vi "Add Logging Group - Right Click.vi"() -> ()   [LabVIEW 2015, in "Waveform Data Logger System Explorer.lvlib"]
uses:
  Waveform Data Logger System Explorer.lvlib
  <vilib>/NI Veristand/Custom Device API/Custom Device Item Ref.ctl
  Shared/Globals/Global GUIDs.vi
  <vilib>/NI VeriStand/Custom Device API/Custom Device API.lvlib
  Shared/Waveform Data Logger Shared.lvlib
panel:
  in  "Node Ptr":T1 format="%.0x"
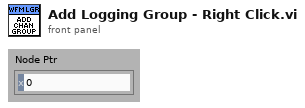
[diagram p1: front panel]
types:
  T1 = typedef "Custom Device API.lvlib/Custom Device Item Ref.ctl" = u64
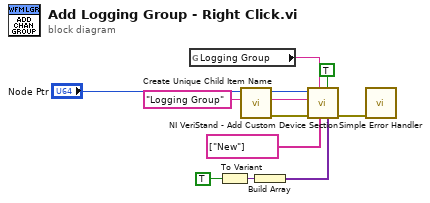
[diagram p0: block diagram]
diagram:
  n1 = global read "Global GUIDs.vi" "Logging Group"() -> (w8:string)
  n2 = To Variant(anything=TRUE) -> (Variant=w4:variant)
  n3 = call "Create Unique Child Item Name.vi"("Name in"="Logging Group", "Parent Item Ref in"="Node Ptr") -> ("error out"=w7:errorcluster, "Unique Name out"=w10:string, "Parent Item Ref out"=w11:T1)  [unwired: 1 in, 6 out]
  n4 = Build Array(w4) -> (w1:variant[])
  n5 = call <vilib>:"NI VeriStand - Add Custom Device Section.vi"("Property Values"=w1, "Highlight? (F)"=TRUE, "Property names"=string[] ["New"], "GUID (Default Section)"=w8, "error in (no error)"=w7, "Section Name"=w10, "Parent Ref in"=w11) -> ("error out"=w5:errorcluster)  [unwired: 4 out]
  n6 = call <vilib>:"Simple Error Handler.vi"("error in (no error)"=w5) -> ()  [unwired: 4 in, 5 out]
